vi "Handle Last Ack Core.vi"(4 "error in (no error)":errorcluster, 6 "Last Ack":refnum<class "Last Ack.lvclass">, 7 "Server in":refnum<class "Server.lvclass">) -> (0 "error out":errorcluster, 3 "Server out":refnum<class "Server.lvclass">)   [LabVIEW 2020, in "Server.lvlib" / "Server.lvclass"]
doc: "(<B>Filename</B>: Actor Framework.lvlib:Actor.lvclass:Handle Last Ack Core.vi)\n\nDefines how the caller actor responds to the Last Ack message from a nested actor. The Last Ack message is the final message a nested actor sends to its caller before it shuts down. The message contains information about the final state of the nested actor.\n\nBy default, this method does nothing except return any error the nested actor sent. A descendant class may override this method to define behavior."
uses:
  Server.lvclass
  Server.lvclass/Server.ctl
  Server Messages/Enable Controls Msg/Enable Controls Msg.lvclass
  <vilib>/ActorFramework/LastAck/Last Ack.lvclass
  Chat Room Model/Chat Room Model Messages/Update Online List Msg/Update Online List Msg.lvclass
  Chat Room Model/Chat Room Model Messages/Update Online Status List Msg/Update Online Status List Msg.lvclass
  e645b656-8103-42f9-8276-0dc2dd4cdd14.vi
  <vilib>/ActorFramework/Actor/Actor.lvclass
  C:/Program Files (x86)/National Instruments/LabVIEW 2020/vi.lib/ActorFramework/Actor/Actor.lvclass
  F:/Gitlab Repository/LabVIEW-Study/10.Top 5 Actor Framework Overrides/Chat Room with Interface/Server/Server/Server.lvclass
  F:/Gitlab Repository/LabVIEW-Study/10.Top 5 Actor Framework Overrides/Chat Room with Interface/Interface/Chat Room Window/Chat Room Window.lvclass
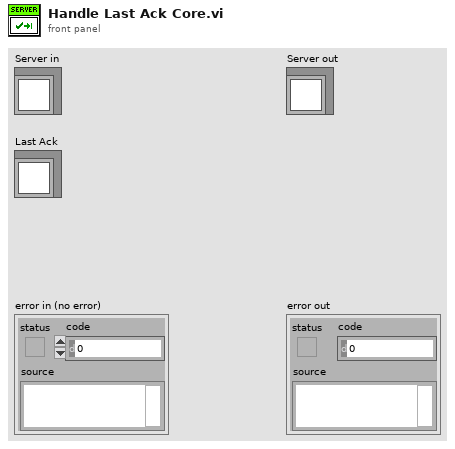
[diagram p1: front panel]
types:
  T1 = enum8{"Enabled", "Disabled", "Disabled and Grayed Out"}
  T2 = typedef "Chat Room Model.lvlib/Chat Room Model.lvclass/User Info.ctl" = cluster{"Name":string, "Status":string}
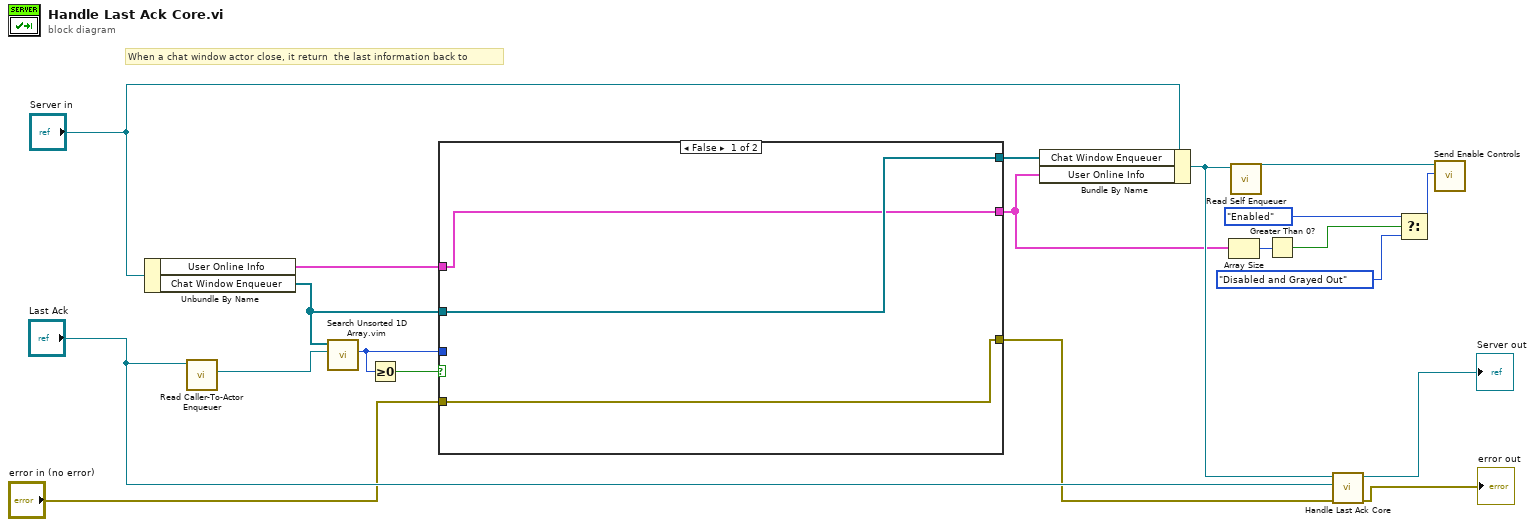
[diagram p0: block diagram]
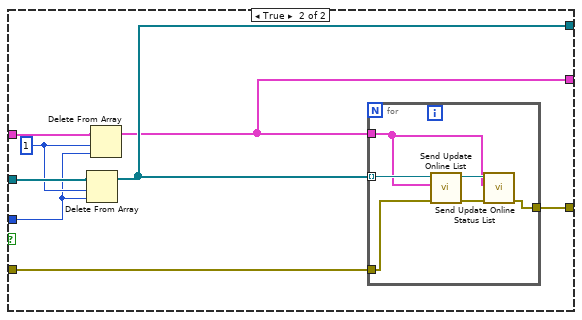
[diagram p2: hidden frame]
diagram:
  # "When a chat window actor close, it return  the last information back to"
  n1 = Unbundle By Name("Server in") -> ("User Online Info"=w13:T2[], "Chat Window Enqueuer"=w15:refnum<class "Message Enqueuer.lvclass">[])
  n2 = call <vilib>:"Read Caller-To-Actor Enqueuer.vi"("Last Ack"="Last Ack") -> ("Caller-to-Actor Enqueuer"=w17:refnum<class "Message Enqueuer.lvclass">)  [unwired: 10 in]
  n3 = call "Search Unsorted 1D Array.vim"("element"=w17, "unsorted 1D array"=w15) -> ("index of element"=w14:i32)  [unwired: 9 in]
  n4 = Greater Or Equal To 0?(x=w14) -> (x >= 0?=w16:bool)
  n5 = case shown="False" w16 {
    tunnel: w15 -> [w23 w31]
    tunnel: w14 -> [_ w26]
    tunnel: w13 -> [w22 w30]
    tunnel: "error in (no error)" -> [w21 w29]
    tunnel: [w22 w25] -> w7
    tunnel: [w23 w28] -> w10
    tunnel: [w21 w24] -> w1
    frame False {
    }
    frame True {
      w27 = 1 ("length")
      n6 = Delete From Array(array=w31, length=w27, index=w26) -> (array with subset deleted=w28:refnum<class "Message Enqueuer.lvclass">[])  [unwired: 1 out]
      n7 = Delete From Array(array=w30, length=w27, index=w26) -> (array with subset deleted=w25:T2[])  [unwired: 1 out]
      n8 = for {
        tunnel: w28 -> [w37] mode=indexing
        tunnel: w29 -> [w35]
        tunnel: w25 -> [w33]
        tunnel: [w32] -> w24
        n9 = call "Send Update Online List.vi"("error in (no error)"=w35, "User Online Info"=w33, "Message Enqueuer"=w37) -> ("error out"=w34:errorcluster, "Message Enqueuer out"=w36:refnum<class "Message Enqueuer.lvclass">)  [unwired: 7 in]
        n10 = call "Send Update Online Status List.vi"("error in (no error)"=w34, "User Online Info"=w33, "Message Enqueuer"=w36) -> ("error out"=w32:errorcluster)  [unwired: 7 in, 1 out]
      }
    }
  }
  n11 = Bundle By Name(cluster="Server in", "Chat Window Enqueuer"=w10, "User Online Info"=w7) -> (w9:refnum<class "Server.lvclass">)
  n12 = Array Size(array=w7) -> (size(s)=w6:i32)
  n13 = call <vilib>:"Read Self Enqueuer.vi"("Actor"=w9) -> ("Self Enqueuer"=w8:refnum<class "Message Enqueuer.lvclass">)  [unwired: 10 in]
  n14 = Greater Than 0?(x=w6) -> (x > 0?=w4:bool)
  n15 = call-parent "Handle Last Ack Core.vi"("error in (no error)"=w1, "Last Ack"="Last Ack", "Actor in"=w9) -> ("error out"=→"error out":errorcluster, "Actor out"=→"Server out":refnum<class "Server.lvclass">)  [unwired: 3 in]
  n16 = Select(t=T1."Enabled" ("Disabled"), s=w4, f=T1."Disabled and Grayed Out" ("Disabled")) -> (s? t:f=w2:T1)
  n17 = call "Send Enable Controls.vi"("Disabled"=w2, "Message Enqueuer"=w8) -> ()  [unwired: 8 in, 2 out]
